vi "Host - Get Module Data.vi"(8 "error in (no error)":errorcluster, 11 "Mod IOVs":refnum<k21>[](array[refnum])) -> (0 "error out":errorcluster, 3 "Modules":T1[](array[typedef]))   [LabVIEW 2011, in "Scan Engine Custom Device.lvlib"]
uses:
  Scan Engine Custom Device.lvlib
  Type Defs/Host - Module.ctl
  Program Files (x86)/National Instruments/LabVIEW 2011/resource/objmgr/cRIO.rc
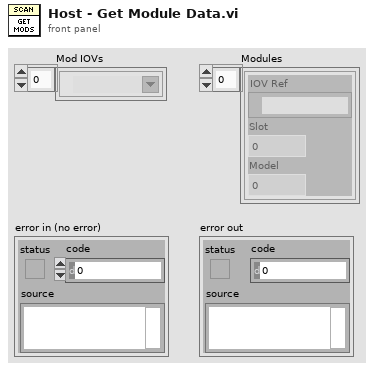
[diagram p1: front panel]
types:
  T1 = typedef "Scan Engine Custom Device.lvlib/Host - Module.ctl" = cluster{"IOV Ref":refnum<k21>, "Slot":u32, "Model":u32}
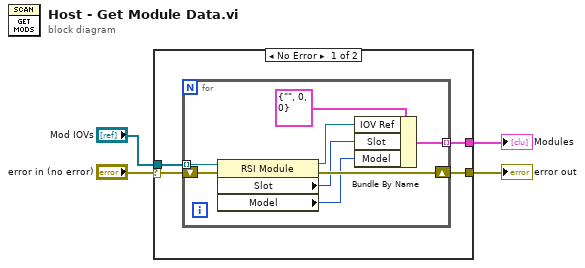
[diagram p0: block diagram]
diagram:
  n1 = case shown="No Error" "error in (no error)" {
    selector: "error in (no error)" -> [w5 w17]
    tunnel: [w8 _] -> w4
    tunnel: [w7 w17] -> w3
    tunnel: "Mod IOVs" -> [w6 _]
    frame No Error {
      n2 = for {
        tunnel: w6 -> [w15] mode=indexing
        shift-right: [w16] -> w7
        shift-left: w5 -> [w14]
        tunnel: [w9] -> w8 mode=indexing
        n3 = property class="RSI Module"(reference=w15, error in=w14) -> (reference out=w12:refnum<k21>, error out=w16:errorcluster, "Slot"=w11:u32, "Model"=w10:u32)
        n4 = Bundle By Name(cluster=T1 {"IOV Ref"="", "Slot"=0, "Model"=0} ("Module"), "IOV Ref"=w12, "Slot"=w11, "Model"=w10) -> (w9:T1)
      }
    }
    frame Error {
    }
  }
  "Modules" <- w4
  "error out" <- w3
